vi "check arm trigger.vi"(9 "always armed?":bool, 10 "armtriggerchannel index":i32, 11 "data table in":T1) -> (2 "Armed?":bool, 3 "Data table out":T1)   [LabVIEW 2013]
uses:
  <vilib>/NI/Tag Bus/table/data table.ctl
  <vilib>/NI/Tag Bus/table/data polymorphs/read one/read Boolean.vi
  <vilib>/NI/Tag Bus/table/data table.lvlib
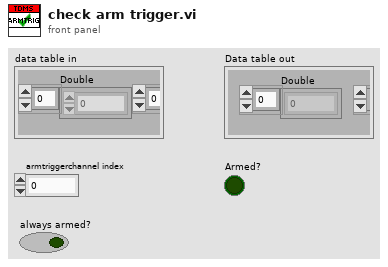
[diagram p1: front panel]
types:
  T1 = typedef "tag bus.lvlib/data table.lvlib/data table.ctl" = cluster{"Double":dbl[], "Single":sgl[], "I64":i64[], "I32":i32[], "I16":i16[], "I8":i8[], "U64":u64[], "U32":u32[], "U16":u16[], "U8":u8[], "Boolean":bool[], "String":string[], "Array of Double":cluster{"DBL Array":dbl[]}[], "Array of Single":cluster{"SGL Array":sgl[]}[], "Array of I64":cluster{"I64 Array":i64[]}[], "Array of I32":cluster{"I32 Array":i32[]}[], "Array of I16":cluster{"I16 Array":i16[]}[], "Array of I8":cluster{"I8 Array":i8[]}[], "Array of U64":cluster{"U64 Array":u64[]}[], "Array of U32":cluster{"U32 Array":u32[]}[], "Array of U16":cluster{"U16 Array":u16[]}[], "Array of U8":cluster{"U8 Array":u8[]}[], "Array of Boolean":cluster{"Boolean Array":bool[]}[], "Array of String":cluster{"String Array":string[]}[]}
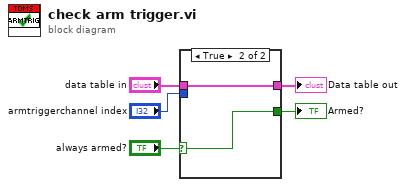
[diagram p0: block diagram]
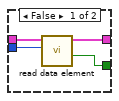
[diagram p2: hidden frame]
diagram:
  n1 = case shown="True" "always armed?" {
    selector: "always armed?" -> [_ w11]
    tunnel: "armtriggerchannel index" -> [w9 _]
    tunnel: [w8 w10] -> w4
    tunnel: "data table in" -> [w7 w10]
    tunnel: [w6 w11] -> w2
    frame False {
      n2 = call-poly <vilib>:"read data element.vi"("index"=w9, "data table in"=w7) -> ("value"=w6:bool, "data table out"=w8:T1)  [unwired: 8 in]
    }
    frame True {
    }
  }
  "Data table out" <- w4
  "Armed?" <- w2
